vi "format_header.vi"(0 "file path (dialog if empty)":path, 7 "values":string) -> (4 "new file path (Not A Path if cancelled)":path)   [LabVIEW 2017, in "ZBOX_IS.lvlib"]
uses:
  ZBOX_IS.lvlib
panel:
  out "String":string
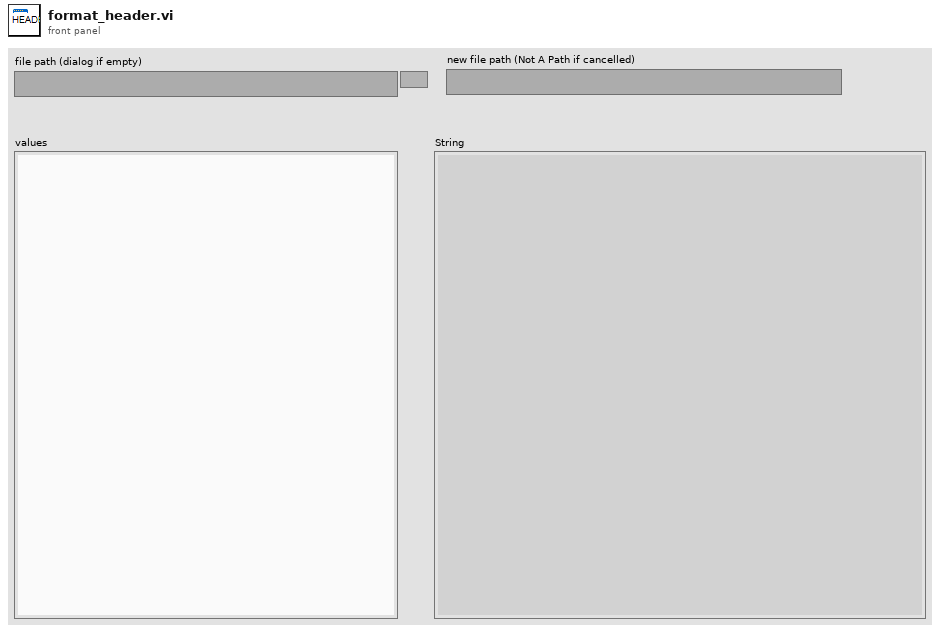
[diagram p1: front panel]
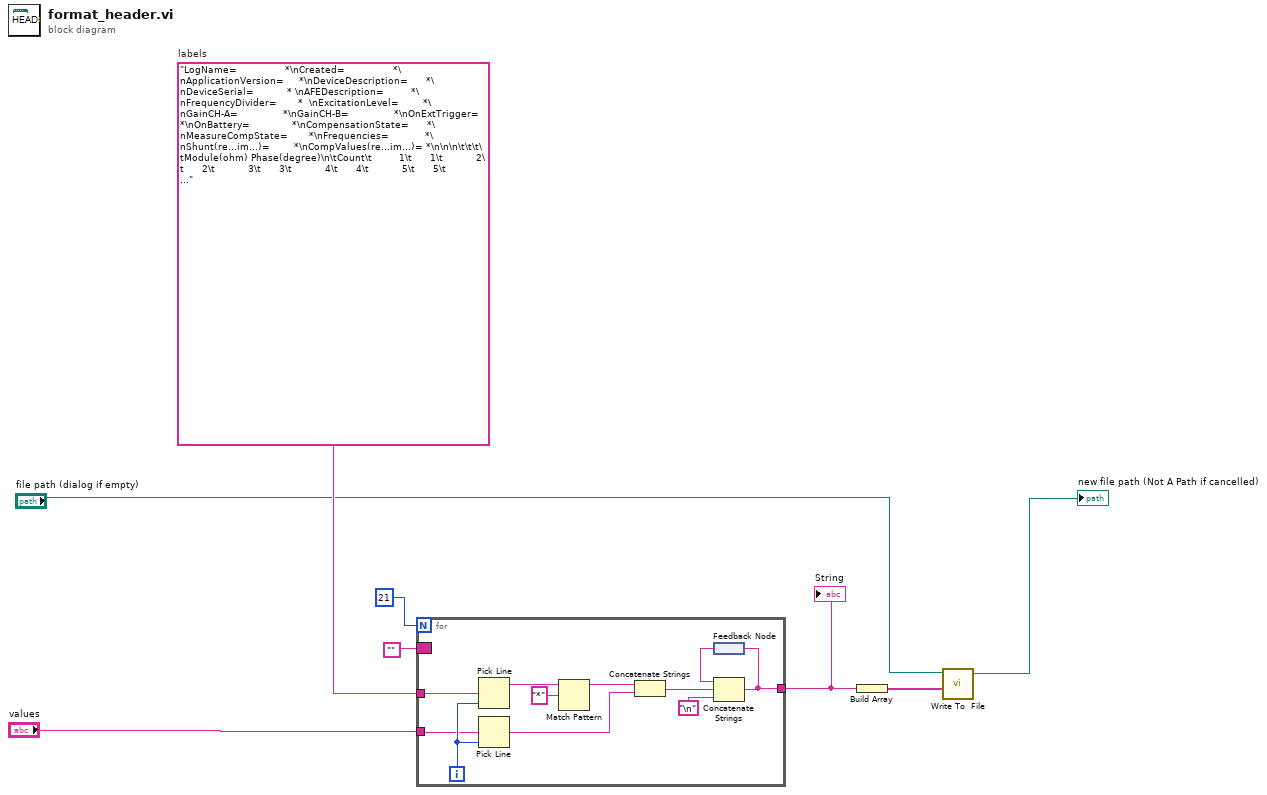
[diagram p0: block diagram]
diagram:
  w8 = "LogName=                *\nCreated=                *\nApplicationVersion=     *\nDeviceDescription=      *\nDeviceSerial=           * \nAFEDescription=         *\nFrequencyDivider=       *  \nExcitationLevel=        *\nGainCH-A=               *\nGainCH-B=               *\nOnExtTrigger=           *\nOnBattery=              *\nCompensationState=      *\nMeasureCompState=       *\nFrequencies=            *\nShunt(re...im...)=        *\nCompValues(re...im...)= *\n\n\n\t\t\t\tModule(ohm) Phase(degree)\n\tCount\t         1\t      1\t           2\t      2\t           3\t      3\t           4\t      4\t           5\t      5\t           6\t      6\t           7\t      7\t           8\t      8\t           9\t      9\t          10\t     10\t          11\t     11\t          12\t     12\t          13\t     13\t          14\t     14\t          15\t     15\tPPeriod(us)\tMax-A\tMin-A\tMax-B\tMin-B\tSysErr\tGPIO\tBattery\tChargeStatus\n"  # labels
  n1 = for {
    N: 21 -> [_]
    tunnel: w8 -> [w19]
    tunnel: [w17] -> w5
    border: "" -> [_]
    tunnel: "values" -> [w9]
    i -> [w11]
    n2 = Pick Line(multi-line string=w19, line index=w11) -> (output string=w15:string)  [unwired: 1 in]
    n3 = Pick Line(multi-line string=w9, line index=w11) -> (output string=w10:string)  [unwired: 1 in]
    n4 = Match Pattern(string=w15, regular expression="*") -> (before substring=w13:string)  [unwired: 1 in, 3 out]
    n5 = Concatenate Strings(w13, w10) -> (w12:string)
    n6 = feedback #1() -> (w18:string)
    n7 = Concatenate Strings(w18, w12, "\n") -> (w17:string)
    n8 = feedback-in #1(w17) -> ()
  }
  "String" <- w5
  n9 = Build Array(w5) -> (w2:string[])
  n10 = call "Write To  File.vi"("1D data"=w2, "file path (dialog if empty)"="file path (dialog if empty)") -> ("new file path (Not A Path if cancelled)"=→"new file path (Not A Path if cancelled)":path)  [unwired: 6 in]
